vi "Timeout Wait.vi"(0 "Seconds to timeout":dbl=300.0 format="%.2f", 1 "Message":string) -> ()   [LabVIEW 2019]
doc: "Waits for the operator to click OK before rearming watchdog timers. This can give an indication if the trip was caused by the watch dog timer or by a magnet deviation. If the OK button is not clicked within 5 minutes, then the VI quits and rearms the watch dog anyway.\nScott Hannahs, NHMFL-FSU, April 1995"
panel:
  in  "OK":bool
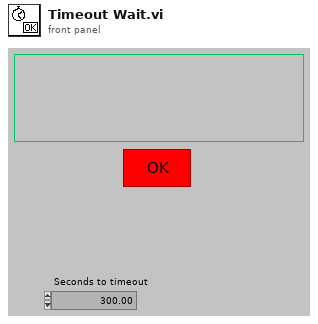
[diagram p1: front panel]
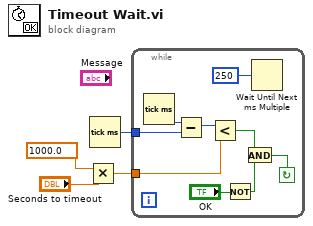
[diagram p0: block diagram]
diagram:
  n1 = Multiply(x=1000.0, y="Seconds to timeout") -> (x*y=w1:dbl)
  n2 = Tick Count (ms)() -> (millisecond timer value=w4:u32)
  n3 = while {
    tunnel: w1 -> [w5]
    tunnel: w4 -> [w11]
    stop <- w6 continue-if-true
    n4 = Tick Count (ms)() -> (millisecond timer value=w12:u32)
    n5 = Subtract(x=w12, y=w11) -> (x-y=w7:u32)
    n6 = Less?(x=w7, y=w5) -> (x < y?=w10:bool)
    n7 = Not(x="OK") -> (.not. x?=w9:bool)
    n8 = And(x=w10, y=w9) -> (x .and. y?=w6:bool)
    n9 = Wait Until Next ms Multiple(millisecond multiple=u32 250) -> ()  [unwired: 1 out]
  }
